vi "Set Setpoint.vi"(7 "Select Channel":i32=1 min=1 max=4 step=1, 8 "error in (no error)":errorcluster, 10 "Setpoint":dbl, 11 "Lakeshore 325 in":refnum<class "Lakeshore 325.lvclass">) -> (0 "error out":errorcluster, 3 "Lakeshore 325 out":refnum<class "Lakeshore 325.lvclass">)   [LabVIEW 2022 SP3, in "Lakeshore 325.lvclass"]
uses:
  Lakeshore 325.lvclass
  Lakeshore 325.lvclass/Lakeshore 325.ctl
  <instrlib>/Lake Shore 325/Lake Shore 325.lvlib
  Temp Control.lvclass
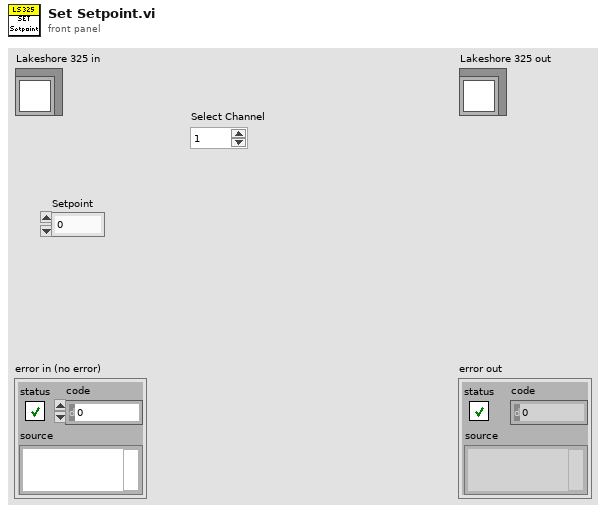
[diagram p1: front panel]
types:
  T1 = typedef "Temp Control.lvclass/Temp Control Parameters.ctl" = cluster{"Mode":u16, "Setpoint":dbl, "Manual Power (%)":dbl, "Control Parameters":cluster{"P":dbl, "I":dbl, "D":u16}, "Heater Range":u16, "Default Range":u16}
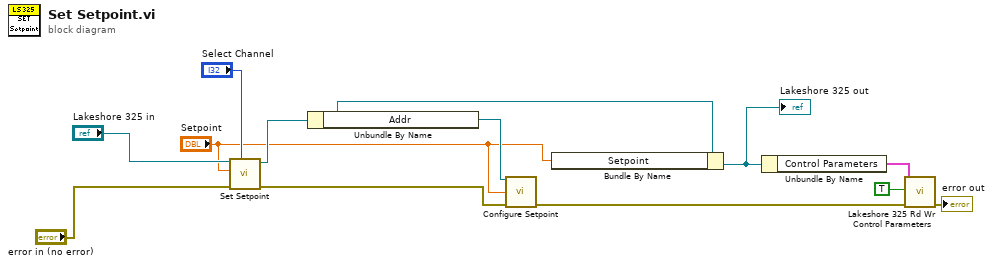
[diagram p0: block diagram]
diagram:
  n1 = call-parent "Set Setpoint.vi"("Select Channel"="Select Channel", "error in (no error)"="error in (no error)", "Setpoint"="Setpoint", "Temp Control in"="Lakeshore 325 in") -> ("error out"=w3:errorcluster, "Temp Control out"=w5:refnum<class "Lakeshore 325.lvclass">)  [unwired: 6 in]
  n2 = Unbundle By Name(w5) -> ("Addr"=w12:refnum<visa-resource-name>)
  n3 = call <instrlib>:"Configure Setpoint.vi"("VISA resource name"=w12, "Setpoint Value (0.0000)"="Setpoint", "error in (no error)"=w3) -> ("error out"=w8:errorcluster)  [unwired: 11 in, 1 out]
  n4 = Bundle By Name(cluster=w5, "Setpoint"="Setpoint") -> (w11:refnum<class "Lakeshore 325.lvclass">)
  "Lakeshore 325 out" <- w11
  n5 = Unbundle By Name(w11) -> ("Control Parameters"=w10:T1)
  n6 = call "Lakeshore 325 Rd Wr Control Parameters.vi"("error in (no error)"=w8, "Write? (F:Read)"=TRUE, "Control Parameters"=w10) -> ("error out"=→"error out":errorcluster)  [unwired: 7 in, 1 out]
